vi "From Variant.vi"(8 "error in (no error)":errorcluster, 10 "Variant":variant, 11 "Abs_I64 Integer in":refnum<class "Abs_I64 Integer.lvclass">) -> (0 "error out":errorcluster, 3 "Abs_I64 Integer out":refnum<class "Abs_I64 Integer.lvclass">)   [LabVIEW 2021, in "Abs_I64 Integer.lvclass"]
uses:
  Abs_I64 Integer.lvclass
  Support/Type.ctl
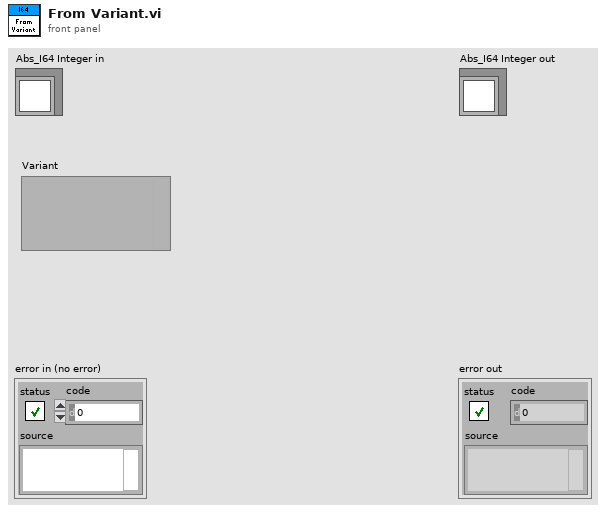
[diagram p1: front panel]
types:
  T1 = typedef "Abs_I64 Integer.lvclass/Type.ctl" = i64
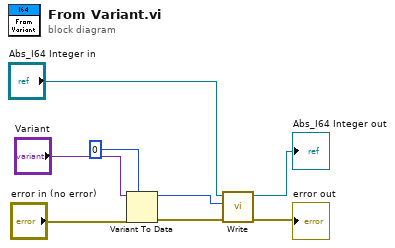
[diagram p0: block diagram]
diagram:
  n1 = Variant To Data(error in="error in (no error)", type=T1 0, Variant="Variant") -> (data=w3:T1, error out=w7:errorcluster)
  n2 = call-dynamic "Write.vi"("error in (no error)"=w7, "Value"=w3, "Double Float.lvclass_340760 in"="Abs_I64 Integer in") -> ("error out"=→"error out":errorcluster, "Double Float.lvclass_340760 out"=→"Abs_I64 Integer out":refnum<class "Abs_I64 Integer.lvclass">)  [unwired: 7 in]
